vi "Read Raw Result.vi"(8 "error in (no error)":errorcluster, 11 "Parameter in":refnum<class "Parameter.lvclass">) -> (0 "error out":errorcluster, 2 "Raw Result":string, 3 "Parameter out":refnum<class "Parameter.lvclass">)   [LabVIEW 2023, in "HAF.lvlib" / "Parameter.lvclass"]
doc: "Returns the unprocessed result."
uses:
  Parameter.lvclass
  Parameter.lvclass/Parameter.ctl
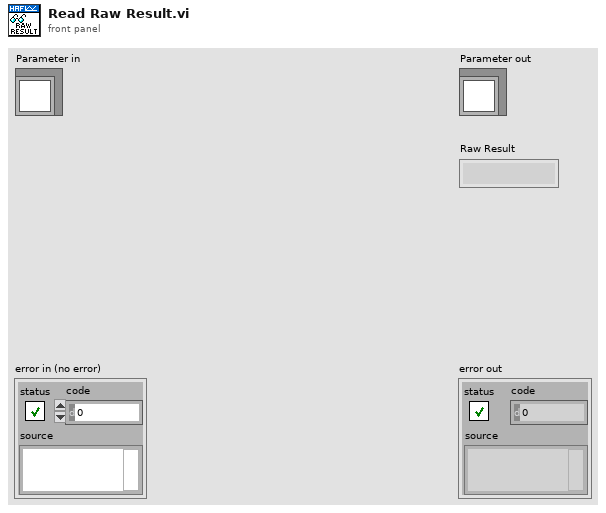
[diagram p1: front panel]
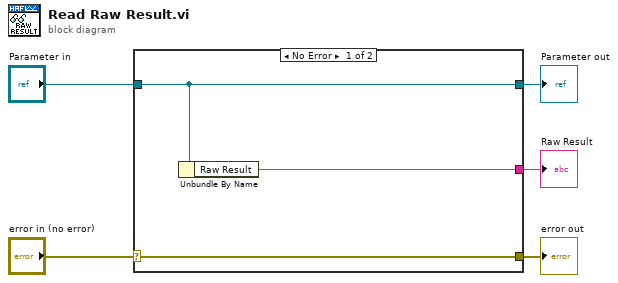
[diagram p0: block diagram]
diagram:
  n1 = case shown="No Error" "error in (no error)" {
    selector: "error in (no error)" -> [w8 w9]
    tunnel: [w8 w9] -> w4
    tunnel: [w7 w10] -> w2
    tunnel: "Parameter in" -> [w7 w10]
    tunnel: [w6 _] -> w1
    frame No Error {
      n2 = Unbundle By Name(w7) -> ("Raw Result"=w6:string)
    }
    frame Error {
    }
  }
  "error out" <- w4
  "Parameter out" <- w2
  "Raw Result" <- w1
